vi "Detect Peak.vi"(4 "Num Samples":dbl=1000.0, 6 "Rate":dbl=10000.0, 8 "error in (no error)":errorcluster, 10 "Threshold":dbl=0.001, 11 "Filtered Signal":dynamicdata(waveform)) -> (0 "error out":errorcluster, 1 "Peak Amplitude":dbl, 2 "Peak Time Stamp":timestamp, 3 "Peak Found?":bool)   [LabVIEW 2016]
doc: "The Detect Peak VI takes the current <b>Num Samples</b> of <b>Filtered Signal</b> that was created at a specific <b>Rate</B> and determines if a peak was found above <b>Threshold</b>.\n\nIf a peak is found in the segment of data the <b>Peak Time Stamp</b> is returned in addition to the <b>Peak Amplitude</b>"
uses:
  <vilib>/Analysis/NI_AAL_SigProc.lvlib
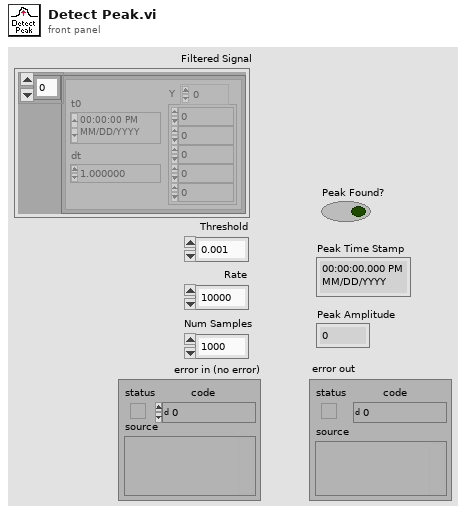
[diagram p1: front panel]
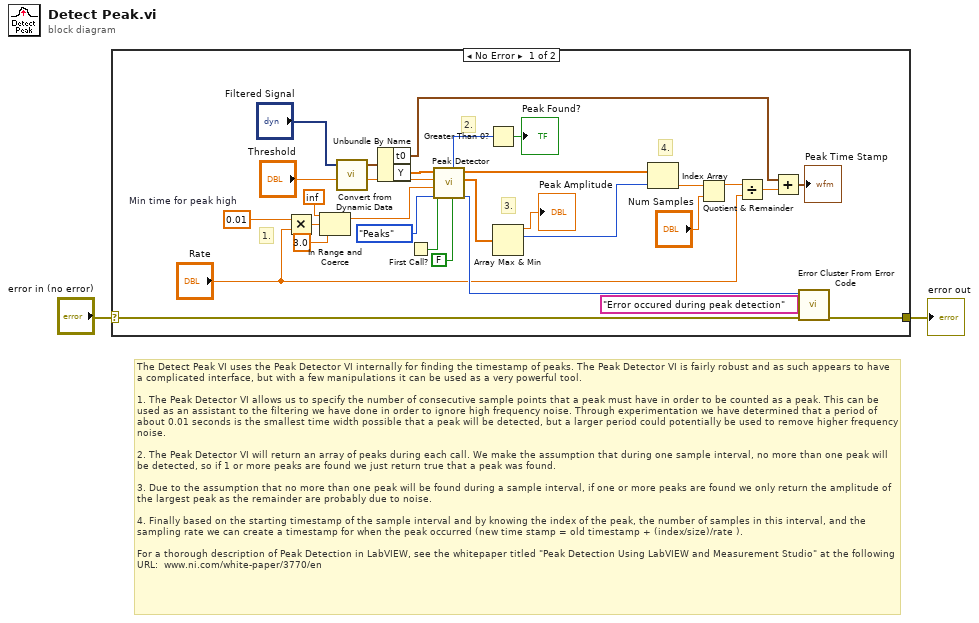
[diagram p0: block diagram]
diagram:
  # "The Detect Peak VI uses the Peak Detector VI internally for finding the timestamp of peaks. The Peak Detector VI is fairly robust and as such appears to have a complicated interface, but with a few manipulations it can be used as a very powerful tool.\n\n1. The Peak Detector VI allows us to specify the number of consecutive sample points that a peak must have in order to be counted as a peak. This can be used as an assistant to the filtering we have done in order to ignore high frequency noise. Through experimentation we have determined that a period of about 0.01 seconds is the smallest time width possible that a peak will be detected, but a larger period could potentially be used to remove higher frequency noise.\n\n2. The Peak Detector VI will return an array of peaks during each call. We make the assumption that during one sample interval, no more than one peak will be detected, so if 1 or more peaks are found we just return true that a peak was found.\n\n3. Due to the assumption that no more than one peak will be found during a sample interval, if one or more peaks are found we only return the amplitude of the largest peak as the remainder are probably due to noise.\n\n4. Finally based on the starting timestamp of the sample interval and by knowing the index of the peak, the number of samples in this interval, and the sampling rate we can create a timestamp for when the peak occurred (new time stamp = old timestamp + (index/size)/rate ).\n\nFor a thorough description of Peak Detection in LabVIEW, see the whitepaper titled \"Peak Detection Using LabVIEW and Measurement Studio\" at the following URL:  www.ni.com/white-paper/3770/en"
  n1 = case shown="No Error" "error in (no error)" {
    selector: "error in (no error)" -> [w16 w32]
    tunnel: [w13 w32] -> w1
    frame No Error {
      w11 = 0.01  # Min time for peak high
      # "4."
      # "3."
      # "2."
      # "1."
      n2 = Multiply(x=w11, y="Rate") -> (x*y=w6:dbl)
      n3 = In Range and Coerce(upper limit=inf, x=w6, lower limit=3.0) -> (coerced(x)=w5:dbl)  [unwired: 1 out]
      n4 = call "Convert from Dynamic Data"("Dynamic Data Type"="Filtered Signal") -> ("Waveform"=w29:waveform(dbl))  [unwired: 3 in]
      n5 = Unbundle By Name(w29) -> ("t0"=w19:timestamp, "Y"=w31:dbl[])
      n6 = First Call?() -> (First Call?: T/F=w27:bool)
      n7 = call <vilib>:"Peak Detector.vi"("end of data (T)"=FALSE, "initialize (T)"=w27, "peaks/valleys"=enum32{"Peaks", "Valleys"}."Peaks", "width"=w5, "threshold"="Threshold", "X"=w31) -> ("error"=w15:i32, "Amplitudes"=w9:dbl[], "Locations"=w28:dbl[], "# found"=w10:i32)  [unwired: 1 in, 1 out]
      n8 = Greater Than 0?(x=w10) -> (x > 0?=→"Peak Found?":bool)
      n9 = Array Max & Min(array=w9) -> (max value=→"Peak Amplitude":dbl, max index (indices)=w8:i32)  [unwired: 2 out]
      n10 = Index Array(array=w28, index=w8) -> (element=w18:dbl)
      n11 = Quotient & Remainder(x=w18, y="Num Samples") -> (x-y*floor(x/y)=w20:dbl)  [unwired: 1 out]
      n12 = Divide(x=w20, y="Rate") -> (x/y=w22:dbl)
      n13 = Add(x=w19, y=w22) -> (x+y=→"Peak Time Stamp":timestamp)
      n14 = call <vilib>:"Error Cluster From Error Code.vi"("error in (no error)"=w16, "error message (\"\")"="Error occured during peak detection" ("error message (\"\")"), "error code (0)"=w15) -> ("error out"=w13:errorcluster)  [unwired: 6 in]
    }
    frame Error {
    }
  }
  "error out" <- w1
